vi "ErrorHandler.vi"(8 "error in":errorcluster, 10 "CameraID":i32, 11 "Caller Enqueuer":refnum<class "Message Enqueuer.lvclass">) -> (0 "error out":errorcluster, 1 "error Details":errorcluster)   [LabVIEW 2019, in "Image Acquisition.lvlib" / "Image Acquisition.lvclass"]
uses:
  Image Acquisition.lvclass
  Camera Controller/Camera Controller Messages/Error Message CC Msg/Error Message CC Msg.lvclass
  <vilib>/ActorFramework/Message Enqueuer/Message Enqueuer.lvclass
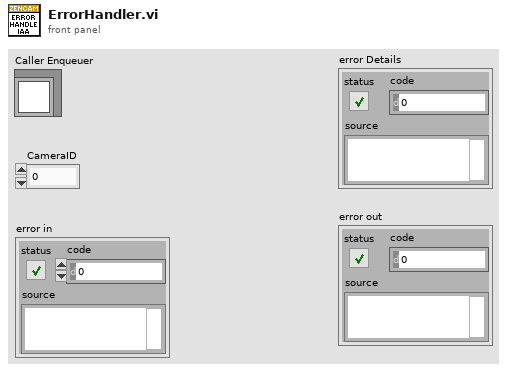
[diagram p1: front panel]
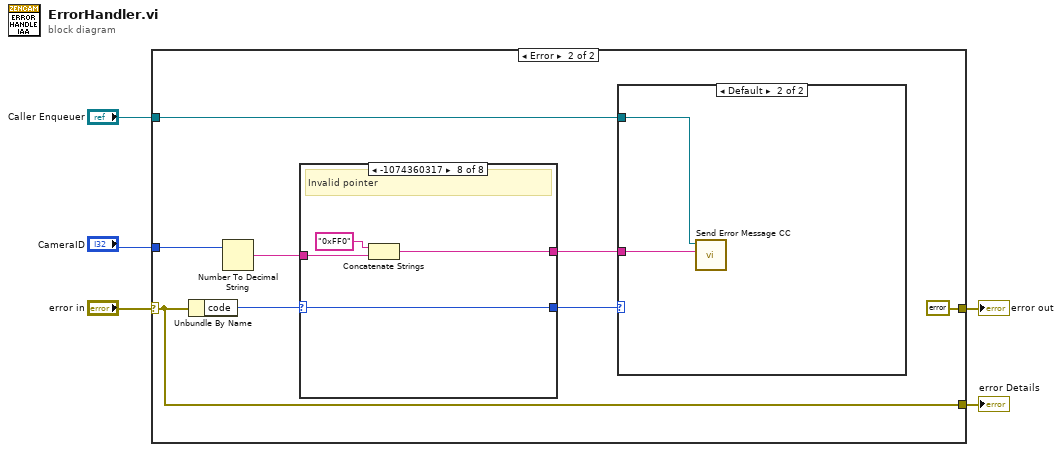
[diagram p0: block diagram]
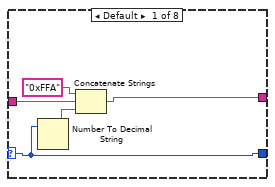
[diagram p4: hidden frame]
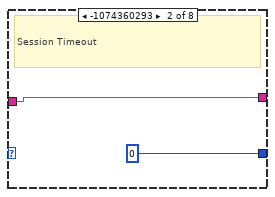
[diagram p5: hidden frame]
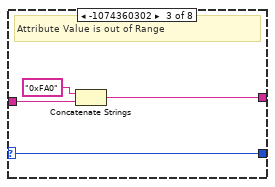
[diagram p6: hidden frame]
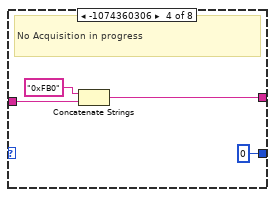
[diagram p7: hidden frame]
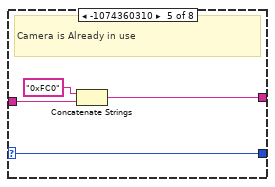
[diagram p8: hidden frame]
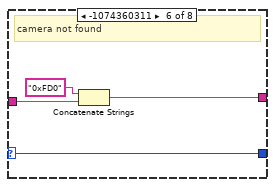
[diagram p9: hidden frame]
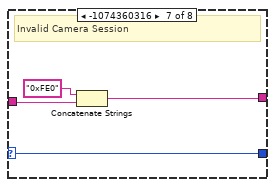
[diagram p10: hidden frame]
diagram:
  n1 = case shown="Error" "error in" {
    selector: "error in" -> [w6 w7]
    tunnel: "CameraID" -> [_ w13]
    tunnel: "Caller Enqueuer" -> [_ w10]
    tunnel: [w6 errorcluster {"status"=FALSE, "code"=0, "source"=""} ("error IO")] -> w2
    tunnel: [w6 w7] -> w1
    frame No Error {
    }
    frame Error {
      n2 = Unbundle By Name(w7) -> ("code"=w14:i32)
      n3 = Number To Decimal String(number=w13) -> (decimal integer string=w12:string)  [unwired: 1 in]
      n4 = case shown="-1074360317" w14 {
        selector: w14 -> [w18 _ w25 _ w33 w37 w41 w45]
        tunnel: w12 -> [w20 w22 w26 w30 w34 w38 w42 w46]
        tunnel: [w18 0 ("code") w25 0 ("code") w33 w37 w41 w45] -> w11
        tunnel: [w19 w22 w24 w29 w32 w36 w40 w44] -> w9
        frame Default {
          n5 = Number To Decimal String(number=w18) -> (decimal integer string=w17:string)  [unwired: 1 in]
          n6 = Concatenate Strings("0xFFA", w20, w17) -> (w19:string)
        }
        frame -1074360293 {
          # "Session Timeout"
        }
        frame -1074360302 {
          # "Attribute Value is out of Range"
          n7 = Concatenate Strings("0xFA0", w26) -> (w24:string)
        }
        frame -1074360306 {
          # "No Acquisition in progress"
          n8 = Concatenate Strings("0xFB0", w30) -> (w29:string)
        }
        frame -1074360310 {
          # "Camera is Already in use"
          n9 = Concatenate Strings("0xFC0", w34) -> (w32:string)
        }
        frame -1074360311 {
          # "camera not found"
          n10 = Concatenate Strings("0xFD0", w38) -> (w36:string)
        }
        frame -1074360316 {
          # "Invalid Camera Session"
          n11 = Concatenate Strings("0xFE0", w42) -> (w40:string)
        }
        frame -1074360317 {
          # "Invalid pointer"
          n12 = Concatenate Strings("0xFF0", w46) -> (w44:string)
        }
      }
      n13 = case shown="Default" w11 {
        tunnel: w10 -> [_ w15]
        tunnel: w9 -> [_ w16]
        frame 0 {
        }
        frame Default {
          n14 = call "Send Error Message CC.vi"("Error Message"=w16, "Message Enqueuer"=w15) -> ()  [unwired: 8 in, 2 out]
        }
      }
    }
  }
  "error out" <- w2
  "error Details" <- w1
